vi "Read Core.vi"(8 "error in (no error)":errorcluster, 9 "Timeout (1s)":dbl[unit]=1.0, 11 "BNT_SLTagConnection in":refnum<class "BNT_SLTagConnection.lvclass">) -> (0 "error out":errorcluster, 1 "timed out":bool, 2 "PV":refnum<class "PV.lvclass">, 3 "BNT_SLTagConnection out":refnum<class "BNT_SLTagConnection.lvclass">)   [LabVIEW 2019, in "BNT_SLTagConnection.lvlib" / "BNT_SLTagConnection.lvclass"]
doc: "Read a process variable."
uses:
  BNT_SLTagConnection.lvclass
  C:/Users/Holger/Documents/LVP/CSPP/CSPP-Template/Packages/CSPP_Core/Classes/CSPP_ProcessVariables/PVConnection/PVConnection.lvclass
  C:/Users/Holger/Documents/LVP/CSPP/CSPP-Template/Packages/CSPP_Core/Classes/CSPP_BaseClasses/Base/CSPP_Base.lvclass
  CSPP_Core/Classes/CSPP_ProcessVariables/ProcessVariable/PV.lvclass
  BNT_SLTagConnection.lvclass/BNT_SLTagConnection.ctl
  <vilib>/Skyline/Tag/Wrapper/Wrapper_class/NI Skyline Tag.lvclass/NI Skyline Tag.ctl
  CSPP_Core/Classes/CSPP_ProcessVariables/PVConnection/PVConnection.lvclass/PVConnection.ctl
  CSPP_Core/Classes/CSPP_ProcessVariables/ProcessVariable/PV.lvclass/PV.ctl
  CSPP_Core/Classes/CSPP_BaseClasses/Base/CSPP_Base.lvclass/CSPP_Base.ctl
  CSPP_Core/Classes/CSPP_ProcessVariables/ProcessVariable/Write Data.vi
  CSPP_Core/Classes/CSPP_ProcessVariables/ProcessVariable/Write Error.vi
  CSPP_Core/Classes/CSPP_ProcessVariables/ProcessVariable/Write Timestamp.vi
  CSPP_Core/Classes/CSPP_ProcessVariables/ProcessVariable/Write status.vi
  CSPP_Core/Classes/CSPP_ProcessVariables/ProcessVariable/Write Quality.vi
  <vilib>/Skyline/Tag/Wrapper/Wrapper_class/Read Tag Path.vi
  <vilib>/Skyline/Tag/Wrapper/Wrapper_class/NI Skyline Tag.lvclass
  <vilib>/Skyline/Tag/Wrapper/Wrapper_class/Read Tag (DBL).vi
  <vilib>/Skyline/Tag/Wrapper/Wrapper_class/Read Tag (String).vi
  <vilib>/Skyline/Tag/Wrapper/Wrapper_class/Read Tag (Timestamp).vi
  <vilib>/Skyline/Tag/Wrapper/Wrapper_class/Read Tag (I32).vi
  <vilib>/Skyline/Tag/Wrapper/Wrapper_class/Read Tag (Boolean).vi
  CSPP_Core/Classes/CSPP_ProcessVariables/PVConnection/PVConnection.lvclass
  CSPP_Core/Libraries/Utilities/CSPP_Utilities.lvlib
  CSPP_Core/Classes/CSPP_BaseClasses/Base/CSPP_Base.lvclass
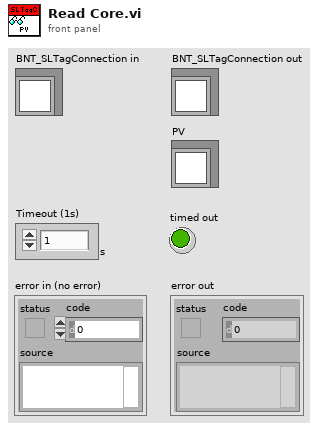
[diagram p1: front panel]
types:
  T1 = cluster{"Read Access":enum8{"Allowed", "Required", "None"}, "Write Access":enum8{"Allowed", "Required", "None"}}
  T2 = typedef "NI Skyline Tag.lvlib/DataType.ctl" = enum32{"Double", "I32", "String", "Boolean", "U64", "Timestamp"}
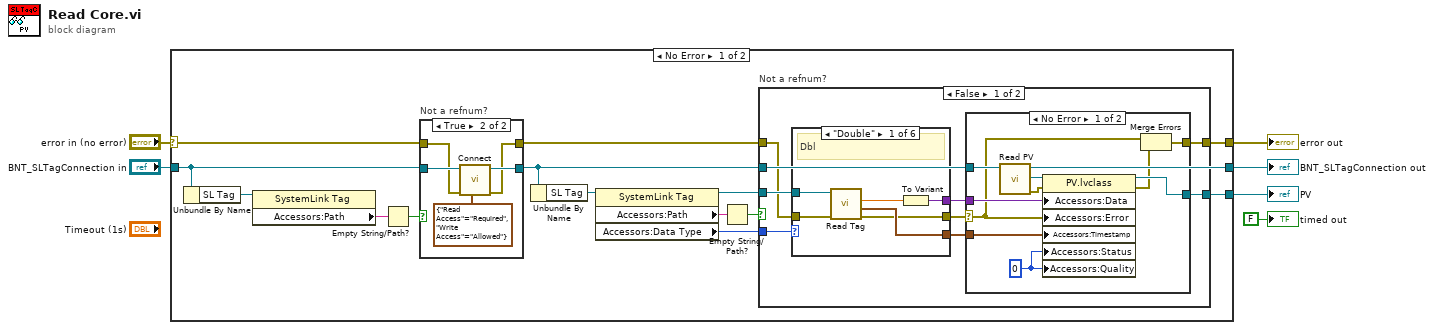
[diagram p0: block diagram]
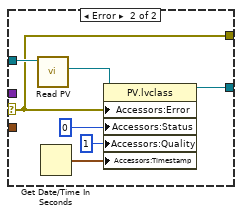
[diagram p3: hidden frame]
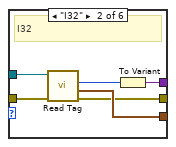
[diagram p4: hidden frame]
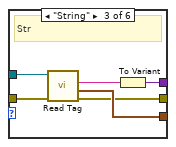
[diagram p5: hidden frame]
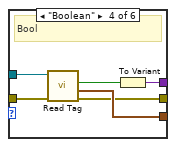
[diagram p6: hidden frame]
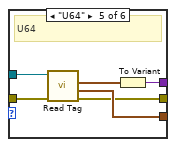
[diagram p7: hidden frame]
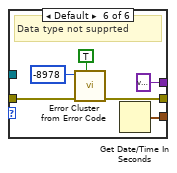
[diagram p8: hidden frame]
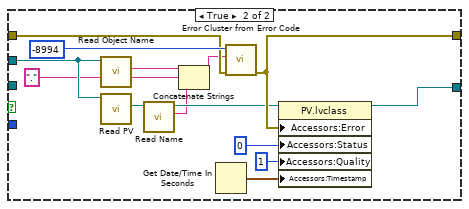
[diagram p9: hidden frame]
diagram:
  n1 = case shown="No Error" "error in (no error)" {
    selector: "error in (no error)" -> [w14 w104]
    tunnel: [w20 w104] -> w3
    tunnel: [w15 w105] -> w4
    tunnel: "BNT_SLTagConnection in" -> [w16 w105]
    tunnel: [w18 _] -> w2
    frame No Error {
      n2 = Unbundle By Name(w16) -> ("SL Tag"=w8:refnum<class "NI Skyline Tag.lvclass">)
      n3 = property class="SystemLink Tag"(reference=w8) -> ("Accessors:Path"=w7:string)  [unwired: 1 in, 2 out]
      n4 = Empty String/Path?(string/path=w7) -> (empty?=w17:bool)
      n5 = case "Not a refnum?" shown="True" w17 {
        tunnel: w16 -> [w21 w27]
        tunnel: [w21 w26] -> w15
        tunnel: w14 -> [w22 w25]
        tunnel: [w22 w24] -> w13
        frame False {
        }
        frame True {
          n6 = call "Connect.vi"("Access (R/W allowed)"=T1 {"Read Access"=enum."Required", "Write Access"=enum."Allowed"}, "Error In"=w25, "PVConnection in"=w27) -> ("Error Out"=w24:errorcluster, "PVConnection out"=w26:refnum<class "BNT_SLTagConnection.lvclass">)  [unwired: 7 in]
        }
      }
      n7 = Unbundle By Name(w15) -> ("SL Tag"=w12:refnum<class "NI Skyline Tag.lvclass">)
      n8 = property class="SystemLink Tag"(reference=w12) -> (reference out=w11:refnum<class "NI Skyline Tag.lvclass">, "Accessors:Path"=w10:string, "Accessors:Data Type"=w9:T2)  [unwired: 1 in, 1 out]
      n9 = Empty String/Path?(string/path=w10) -> (empty?=w19:bool)
      n10 = case "Not a refnum?" shown="False" w19 {
        tunnel: w11 -> [w36 _]
        tunnel: w13 -> [w35 w102]
        tunnel: [w30 w100] -> w20
        tunnel: w15 -> [w34 w94]
        tunnel: [w31 w101] -> w18
        tunnel: w9 -> [w28 _]
        frame False {
          n11 = case shown="\"Double\"" w28 {
            tunnel: w36 -> [w59 w65 w71 w77 w83 _]
            tunnel: w35 -> [w58 w64 w70 w76 w82 w84]
            tunnel: [w54 w60 w66 w72 w78 variant ("Variant")] -> w33
            tunnel: [w56 w62 w68 w74 w80 w89] -> w32
            tunnel: [w55 w61 w67 w73 w79 w85] -> w29
            frame "Double" {
              # "Dbl"
              n12 = call-poly <vilib>:"Read Tag.vi"("error in (no error)"=w58, "tag in"=w59) -> ("error out"=w55:errorcluster, "time stamp"=w56:timestamp, "value"=w57:dbl)  [unwired: 5 in, 2 out]
              n13 = To Variant(anything=w57) -> (Variant=w54:variant)
            }
            frame "I32" {
              # "I32"
              n14 = call-poly <vilib>:"Read Tag.vi"("error in (no error)"=w64, "tag in"=w65) -> ("error out"=w61:errorcluster, "time stamp"=w62:timestamp, "value"=w63:i32)  [unwired: 5 in, 2 out]
              n15 = To Variant(anything=w63) -> (Variant=w60:variant)
            }
            frame "String" {
              # "Str"
              n16 = call-poly <vilib>:"Read Tag.vi"("error in (no error)"=w70, "tag in"=w71) -> ("error out"=w67:errorcluster, "time stamp"=w68:timestamp, "value"=w69:string)  [unwired: 5 in, 2 out]
              n17 = To Variant(anything=w69) -> (Variant=w66:variant)
            }
            frame "Boolean" {
              # "Bool"
              n18 = call-poly <vilib>:"Read Tag.vi"("error in (no error)"=w76, "tag in"=w77) -> ("error out"=w73:errorcluster, "time stamp"=w74:timestamp, "value"=w75:bool)  [unwired: 5 in, 2 out]
              n19 = To Variant(anything=w75) -> (Variant=w72:variant)
            }
            frame "U64" {
              # "U64"
              n20 = call-poly <vilib>:"Read Tag.vi"("error in (no error)"=w82, "tag in"=w83) -> ("error out"=w79:errorcluster, "time stamp"=w80:timestamp, "value"=w81:timestamp)  [unwired: 5 in, 2 out]
              n21 = To Variant(anything=w81) -> (Variant=w78:variant)
            }
            frame Default {
              # "Data type not supprted"
              n22 = call "Error Cluster from Error Code.vi"("show call chain? (False)"=TRUE, "Error In"=w84, "Error Code (0)"=-8978 ("error code (0)")) -> ("Error Out"=w85:errorcluster)  [unwired: 8 in]
              n23 = Get Date/Time In Seconds() -> (seconds since 1Jan1904=w89:timestamp)
            }
          }
          n24 = case shown="No Error" w29 {
            selector: w29 -> [w37 w48]
            tunnel: w34 -> [w46 w53]
            tunnel: w33 -> [w45 _]
            tunnel: w32 -> [w44 _]
            tunnel: [w42 w47] -> w31
            tunnel: [w38 w48] -> w30
            frame No Error {
              w43 = u32 0 ("status")
              n25 = call "Read PV.vi"("PVConnection in"=w46) -> ("error out"=w40:errorcluster, "PV"=w41:refnum<class "PV.lvclass">)  [unwired: 8 in, 1 out]
              n26 = property class="PV.lvclass"(reference=w41, error in=w40, "Accessors:Data"=w45, "Accessors:Error"=w37, "Accessors:Timestamp"=w44, "Accessors:Status"=w43, "Accessors:Quality"=w43) -> (reference out=w42:refnum<class "PV.lvclass">, error out=w39:errorcluster)
              n27 = Merge Errors(w37, w39) -> (w38:errorcluster)
            }
            frame Error {
              n28 = call "Read PV.vi"("PVConnection in"=w53) -> ("PV"=w49:refnum<class "PV.lvclass">)  [unwired: 8 in, 2 out]
              n29 = Get Date/Time In Seconds() -> (seconds since 1Jan1904=w52:timestamp)
              n30 = property class="PV.lvclass"(reference=w49, "Accessors:Error"=w48, "Accessors:Status"=u32 0 ("status"), "Accessors:Quality"=u64 1 ("quality"), "Accessors:Timestamp"=w52) -> (reference out=w47:refnum<class "PV.lvclass">)  [unwired: 1 in, 1 out]
            }
          }
        }
        frame True {
          n31 = call "Read Object Name.vi"("Base in"=w94) -> ("Object Name"=w93:string)  [unwired: 8 in, 2 out]
          n32 = call "Read PV.vi"("PVConnection in"=w94) -> ("PV"=w96:refnum<class "PV.lvclass">)  [unwired: 8 in, 2 out]
          n33 = call "Read Name.vi"("PV in"=w96) -> ("Name"=w91:string, "PV out"=w95:refnum<class "PV.lvclass">)  [unwired: 8 in, 1 out]
          n34 = Concatenate Strings(w93, "." ("string"), w91) -> (w90:string)
          n35 = Get Date/Time In Seconds() -> (seconds since 1Jan1904=w97:timestamp)
          n36 = call "Error Cluster from Error Code.vi"("Error In"=w102, "Error Message (\"\")"=w90, "Error Code (0)"=-8994 ("error code (0)")) -> ("Error Out"=w100:errorcluster)  [unwired: 8 in]
          n37 = property class="PV.lvclass"(reference=w95, "Accessors:Error"=w100, "Accessors:Status"=u32 0 ("status"), "Accessors:Quality"=u64 1 ("quality"), "Accessors:Timestamp"=w97) -> (reference out=w101:refnum<class "PV.lvclass">)  [unwired: 1 in, 1 out]
        }
      }
    }
    frame Error {
    }
  }
  "error out" <- w3
  "BNT_SLTagConnection out" <- w4
  "PV" <- w2
  "timed out" <- FALSE ("timed out")
